vi "GWInstek  GDM8351 Acquire Software Triggered Multiple.vi"() -> ()   [LabVIEW 2021]
doc: "This example shows how to configure a measurement, set up triggering, trigger a measurement, and retrieve a measurement. It shows how to use the low-level Data VIs to retrieve data from the DMM."
uses:
  <instrlib>/GWInstek  GDM8351/GWInstek  GDM8351.lvlib
panel:
  in  "Baud Rate (115200)":u32(ring)=115200 items=["9600"=9600, "19200"=19200, "38400"=38400, "57600"=57600, "115200"=115200]
  in  "Function (0: DC Volts)":u16(ring) items=["DC Volts", "AC Volts", "DC+AC Volts", "DC Current", "AC Current", "DC+AC Current", "2-Wire Resistance", "4-Wire Resistance", "Frequency", "Period", "Continuity", "Diode", "Temperature", "Capacitance"]
  in  "Sample Count (10)":i32=10 format="%#.6g"
  out "Waveform Chart":dbl(graph)
  in  "VISA resource name":refnum<visa-resource-name>
  # "(c) 2014 GWInstek.  ALL RIGHTS RESERVED."
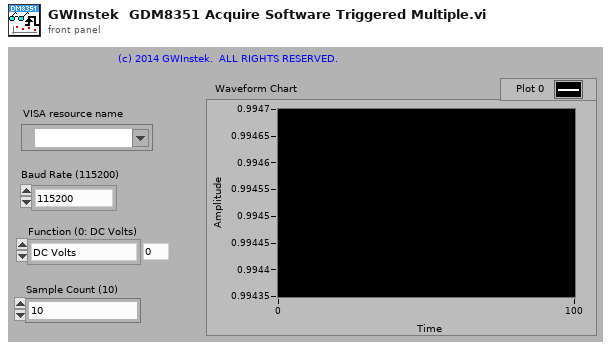
[diagram p1: front panel]
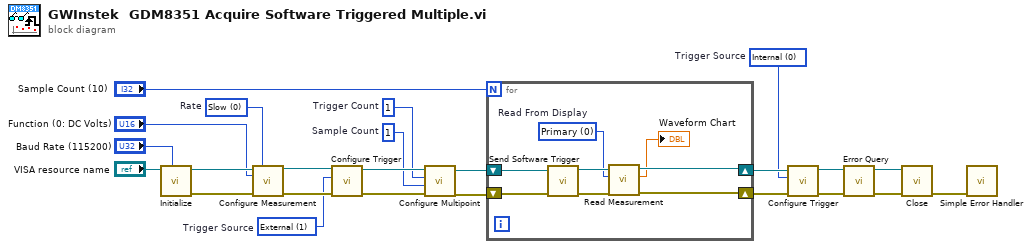
[diagram p0: block diagram]
diagram:
  w1 = u16 0 items=["Slow", "Mid", "Fast"]  # Rate
  w3 = 1  # Sample Count
  w4 = 1  # Trigger Count
  w5 = u16 0 items=["Internal", "External"]  # Trigger Source
  w14 = u16 1 items=["Internal", "External"]  # Trigger Source
  n1 = call <instrlib>:"Initialize.vi"("Baud Rate (115200)"="Baud Rate (115200)", "VISA resource name"="VISA resource name") -> ("error out"=w22:errorcluster, "VISA resource name out"=w23:refnum<visa-resource-name>)  [unwired: 8 in]
  n2 = call <instrlib>:"Configure Measurement.vi"("VISA resource name"=w23, "Rate (0: Slow)"=w1, "Function (0: DC Volts)"="Function (0: DC Volts)", "error in (no error)"=w22) -> ("VISA resource name out"=w21:refnum<visa-resource-name>, "error out"=w20:errorcluster)  [unwired: 10 in]
  n3 = call <instrlib>:"Configure Trigger.vi"("error in (no error)"=w20, "Trigger Source (0: Internal)"=w14, "VISA resource name"=w21) -> ("error out"=w18:errorcluster, "VISA resource name out"=w19:refnum<visa-resource-name>)  [unwired: 7 in]
  n4 = call <instrlib>:"Configure Multipoint.vi"("error in (no error)"=w18, "Sample Count (1)"=w3, "Trigger Count (1)"=w4, "VISA resource name"=w19) -> ("error out"=w10:errorcluster, "VISA resource name out"=w11:refnum<visa-resource-name>)  [unwired: 6 in]
  n5 = for {
    N: "Sample Count (10)" -> [_]
    shift-right: [w27] -> w6
    shift-left: w10 -> [w31]
    shift-right: [w28] -> w7
    shift-left: w11 -> [w32]
    w26 = u16 0 items=["Primary", "Secondary", "Both"]  # Read From Display
    n6 = call <instrlib>:"Send Software Trigger.vi"("error in (no error)"=w31, "VISA resource name"=w32) -> ("error out"=w29:errorcluster, "VISA resource name out"=w30:refnum<visa-resource-name>)  [unwired: 8 in]
    n7 = call <instrlib>:"Read Measurement.vi"("error in (no error)"=w29, "Display (0: Primary)"=w26, "VISA resource name"=w30) -> ("error out"=w27:errorcluster, "Primary Measurement"=→"Waveform Chart":dbl, "VISA resource name out"=w28:refnum<visa-resource-name>)  [unwired: 5 in, 1 out]
  }
  n8 = call <instrlib>:"Configure Trigger.vi"("error in (no error)"=w6, "Trigger Source (0: Internal)"=w5, "VISA resource name"=w7) -> ("error out"=w9:errorcluster, "VISA resource name out"=w8:refnum<visa-resource-name>)  [unwired: 7 in]
  n9 = call <instrlib>:"Error Query.vi"("error in (no error)"=w9, "VISA resource name"=w8) -> ("error out"=w15:errorcluster, "VISA resource name out"=w16:refnum<visa-resource-name>)  [unwired: 6 in, 2 out]
  n10 = call <instrlib>:"Close.vi"("error in (no error)"=w15, "VISA resource name"=w16) -> ("error out"=w17:errorcluster)  [unwired: 9 in]
  n11 = call <vilib>:"Simple Error Handler.vi"("error in (no error)"=w17) -> ()  [unwired: 4 in, 5 out]
